vi "Tester Events FGV.vi"(8 "error in":errorcluster, 11 "Action":T1) -> (0 "error out":errorcluster, 3 "User Events":T2)   [LabVIEW 2024, in "Tester InterComm.lvlib"]
uses:
  Tester InterComm.lvlib
  Tester Events.ctl
  General Actions.ctl
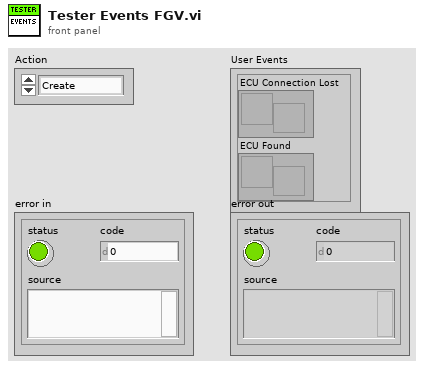
[diagram p1: front panel]
types:
  T1 = typedef "Tester InterComm.lvlib/General Actions.ctl" = enum16{"Create", "Get", "Destroy"}
  T2 = typedef "Tester InterComm.lvlib/Tester Events.ctl" = cluster{"ECU Connection Lost":refnum<user-event>, "ECU Found":refnum<user-event>}
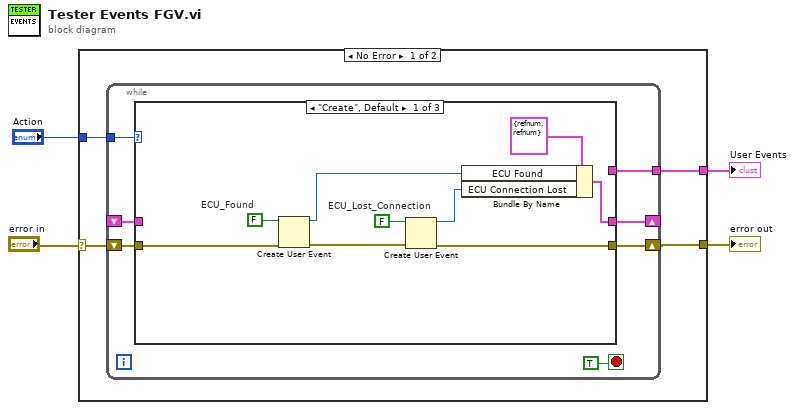
[diagram p0: block diagram]
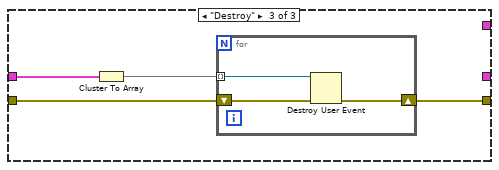
[diagram p3: hidden frame]
diagram:
  n1 = case shown="No Error" "error in" {
    selector: "error in" -> [w7 w34]
    tunnel: "Action" -> [w8 _]
    tunnel: [w6 _] -> w2
    tunnel: [w5 w34] -> w1
    frame No Error {
      n2 = while {
        tunnel: w8 -> [w14]
        shift-right: [w12] -> w5
        shift-left: w7 -> [w13]
        shift-right: [w11] -> _
        shift-left: _ -> [w10]
        tunnel: [w9] -> w6
        stop <- TRUE stop-if-true
        n3 = case shown="\"Create\", Default" w14 {
          tunnel: w13 -> [w18 w25 w30]
          tunnel: [w23 w25 w29] -> w12
          tunnel: [w20 w26 _] -> w11
          tunnel: w10 -> [_ w26 w28]
          tunnel: [_ w26 _] -> w9
          frame "Create", Default {
            w19 = FALSE  # ECU_Found
            w24 = FALSE  # ECU_Lost_Connection
            n4 = Create User Event(user event datatype=w19, error in=w18) -> (user event=w16:refnum<user-event>, error out=w17:errorcluster)
            n5 = Create User Event(user event datatype=w24, error in=w17) -> (user event=w21:refnum<user-event>, error out=w23:errorcluster)
            n6 = Bundle By Name(cluster=T2 {"ECU Connection Lost"=refnum, "ECU Found"=refnum} ("User Events"), "ECU Found"=w16, "ECU Connection Lost"=w21) -> (w20:T2)
          }
          frame "Get" {
          }
          frame "Destroy" {
            n7 = Cluster To Array(cluster=w28) -> (array=w27:refnum<user-event>[])
            n8 = for {
              shift-right: [w32] -> w29
              shift-left: w30 -> [w33]
              tunnel: w27 -> [w31] mode=indexing
              n9 = Destroy User Event(user event=w31, error in=w33) -> (error out=w32:errorcluster)
            }
          }
        }
      }
    }
    frame Error {
    }
  }
  "User Events" <- w2
  "error out" <- w1
